vi "tcp-ip-test.vi"() -> ()   [LabVIEW 2017]
panel:
  out "error out":errorcluster
  out "data out":string
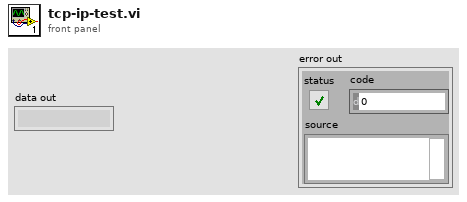
[diagram p1: front panel]
types:
  T1 = enum16{"Standard", "Buffered", "CRLF", "Immediate"}
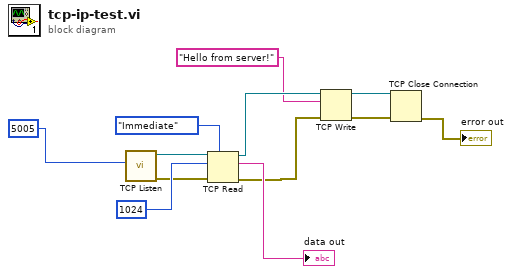
[diagram p0: block diagram]
diagram:
  n1 = call <vilib>:"TCP Listen.vi"("port"=u16 5005 ("remote port or service name")) -> ("error out"=w8:errorcluster, "connection ID"=w11:refnum<k5>)  [unwired: 6 in, 3 out]
  n2 = TCP Read(connection ID=w11, bytes to read=1024, error in (no error)=w8, 7:T1."Immediate" ("mode (standard)")) -> (connection ID out=w7:refnum<k5>, data out=→"data out":string, error out=w5:errorcluster)  [unwired: 1 in]
  n3 = TCP Write(connection ID=w7, data in="Hello from server!", error in (no error)=w5) -> (connection ID out=w2:refnum<k5>, error out=w4:errorcluster)  [unwired: 1 in, 1 out]
  n4 = TCP Close Connection(connection ID=w2, error in (no error)=w4) -> (error out=→"error out":errorcluster)  [unwired: 1 in, 1 out]
